vi "Get Alarm State.vi"(11 "Pump_1AI_1DO_2DI in":refnum<class "Engine_1DO_2DI.lvclass">) -> (2 "Alarm State":bool)   [LabVIEW 2019, in "Engine_1DO_2DI.lvclass"]
uses:
  Engine_1DO_2DI.lvclass
  Engine_1DO_2DI.lvclass/Engine_1DO_2DI.ctl
  Sig_DA_class/Sig_DA.lvclass/Sig_DA.ctl
  Sig_DA_class/Sig_DA.lvclass
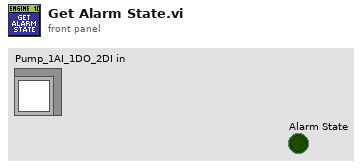
[diagram p1: front panel]
types:
  T1 = typedef "bool_data.ctl" = cluster{"CURR":bool, "RAW_PREV":bool, "millisecond timer value":u32}
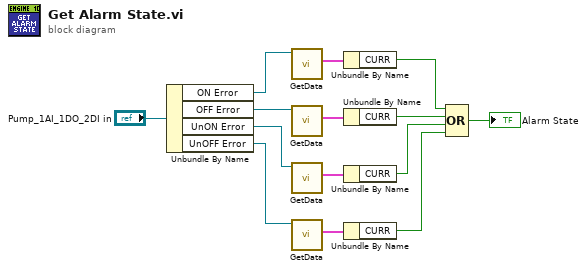
[diagram p0: block diagram]
diagram:
  n1 = Unbundle By Name("Pump_1AI_1DO_2DI in") -> ("ON Error"=w13:refnum<class "Sig_DA.lvclass">, "OFF Error"=w8:refnum<class "Sig_DA.lvclass">, "UnON Error"=w7:refnum<class "Sig_DA.lvclass">, "UnOFF Error"=w6:refnum<class "Sig_DA.lvclass">)
  n2 = call "GetData.vi"("Sig_DA in"=w13) -> ("data"=w12:T1)  [unwired: 10 in]
  n3 = call "GetData.vi"("Sig_DA in"=w8) -> ("data"=w11:T1)  [unwired: 10 in]
  n4 = call "GetData.vi"("Sig_DA in"=w7) -> ("data"=w10:T1)  [unwired: 10 in]
  n5 = call "GetData.vi"("Sig_DA in"=w6) -> ("data"=w9:T1)  [unwired: 10 in]
  n6 = Unbundle By Name(w12) -> ("CURR"=w5:bool)
  n7 = Unbundle By Name(w11) -> ("CURR"=w4:bool)
  n8 = Unbundle By Name(w10) -> ("CURR"=w3:bool)
  n9 = Unbundle By Name(w9) -> ("CURR"=w2:bool)
  n10 = Compound Arithmetic op=OR(w5, w4, w3, w2) -> (→"Alarm State":bool)
